vi "Get Wheel Information_Omnidirectional.vi"(8 "error in (no error)":errorcluster, 11 "omnidirectional wheel in":refnum<class "NI_Robotics_Omnidirectional Wheel.lvclass">) -> (0 "error out":errorcluster, 1 "wheel name":string, 2 "wheel parameters":T1={"wheel radius"=1.0, "gear ratio"=1.0, "forward rotation direction"=0} {"forward rotation direction" items=["Clockwise", "Counterclockwise"]}, 3 "omnidirectional wheel out":refnum<class "NI_Robotics_Omnidirectional Wheel.lvclass">, 4 "motor communication":refnum<class "NI_Robotics_Motor Communication.lvclass">)   [LabVIEW 2017, in "NI_Robotics_Omnidirectional Wheel.lvclass"]
doc: "Returns information, such as <B>wheel radius</B> and <B>gear ratio</B>, for the wheel you specify. You must manually select the polymorphic instance to use."
uses:
  <vilib>/robotics/Steering/Omnidirectional Wheel/NI_Robotics_Omnidirectional Wheel.lvclass
  c:/Program Files (x86)/National Instruments/LabVIEW 2017/vi.lib/robotics/Steering/Wheel/NI_Robotics_Wheel.lvclass
  <vilib>/robotics/Steering/Wheel/Wheel Parameters.ctl
  <vilib>/robotics/Steering/Wheel/Rotation Direction.ctl
  <vilib>/robotics/Actuation/Motor Communication/NI_Robotics_Motor Communication.lvclass
  <vilib>/robotics/Steering/Wheel/NI_Robotics_Wheel.lvclass/NI_Robotics_Wheel.ctl
  <vilib>/robotics/Steering/Wheel/NI_Robotics_Wheel.lvclass
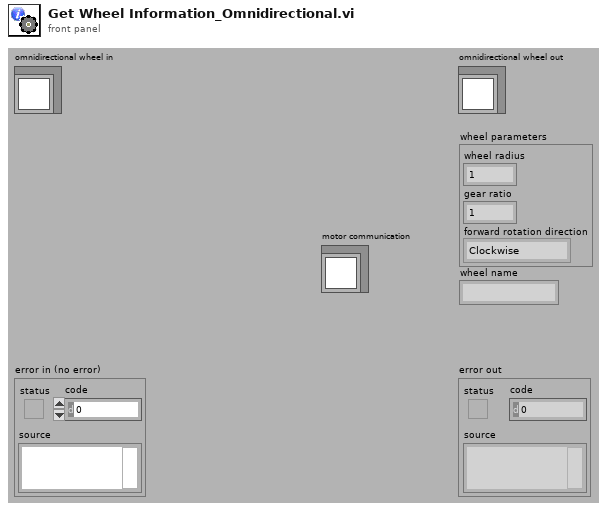
[diagram p1: front panel]
types:
  T1 = typedef "NI_Robotics_Wheel.lvclass/Wheel Parameters.ctl" = cluster{"wheel radius":dbl, "gear ratio":dbl, "forward rotation direction":T2}
  T2 = typedef "NI_Robotics_Wheel.lvclass/Rotation Direction.ctl" = u16
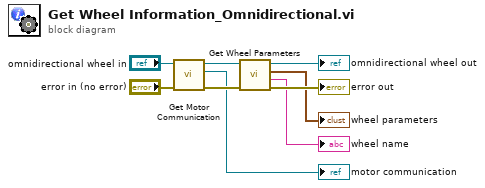
[diagram p0: block diagram]
diagram:
  n1 = call <vilib>:"Get Motor Communication.vi"("error in (no error)"="error in (no error)", "wheel in"="omnidirectional wheel in") -> ("error out"=w6:errorcluster, "motor communication"=→"motor communication":refnum<class "NI_Robotics_Motor Communication.lvclass">, "wheel out"=w9:refnum<class "NI_Robotics_Omnidirectional Wheel.lvclass">)  [unwired: 7 in]
  n2 = call <vilib>:"Get Wheel Parameters.vi"("error in (no error)"=w6, "wheel in"=w9) -> ("error out"=→"error out":errorcluster, "wheel name"=→"wheel name":string, "wheel parameters"=→"wheel parameters":T1, "wheel out"=→"omnidirectional wheel out":refnum<class "NI_Robotics_Omnidirectional Wheel.lvclass">)  [unwired: 6 in]
